vi "FunctionGenerator_Add_Value.vi"(9 "Y Value":dbl, 10 "X Value":dbl, 11 "in FUNCTION_GENERATOR":T1) -> (3 "out FUNCTION_GENERATOR":T1)   [LabVIEW 2019, in "Trajectory_Library.lvlib"]
doc: "Insert new X, Y pair into an existing Function Generator data cluster. If the X values matches an existing X value, the new X and Y values replaces the old values.\n\nInputs:\n - In Function Generator -- Function generator data cluster\n - X -- X value\n - Y -- Y value\n\nOutputs:\n - out Function Generator -- updated data structure"
uses:
  Trajectory_Library.lvlib
  TypeDef/FUNCTION_GENERATOR.ctl
  <vilib>/gmath/NI_Gmath.lvlib
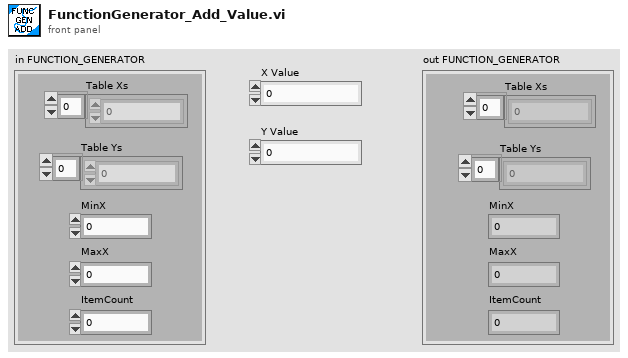
[diagram p1: front panel]
types:
  T1 = typedef "Trajectory_Library.lvlib/FUNCTION_GENERATOR.ctl" = cluster{"Table Xs":dbl[], "Table Ys":dbl[], "MinX":dbl, "MaxX":dbl, "ItemCount":i32}
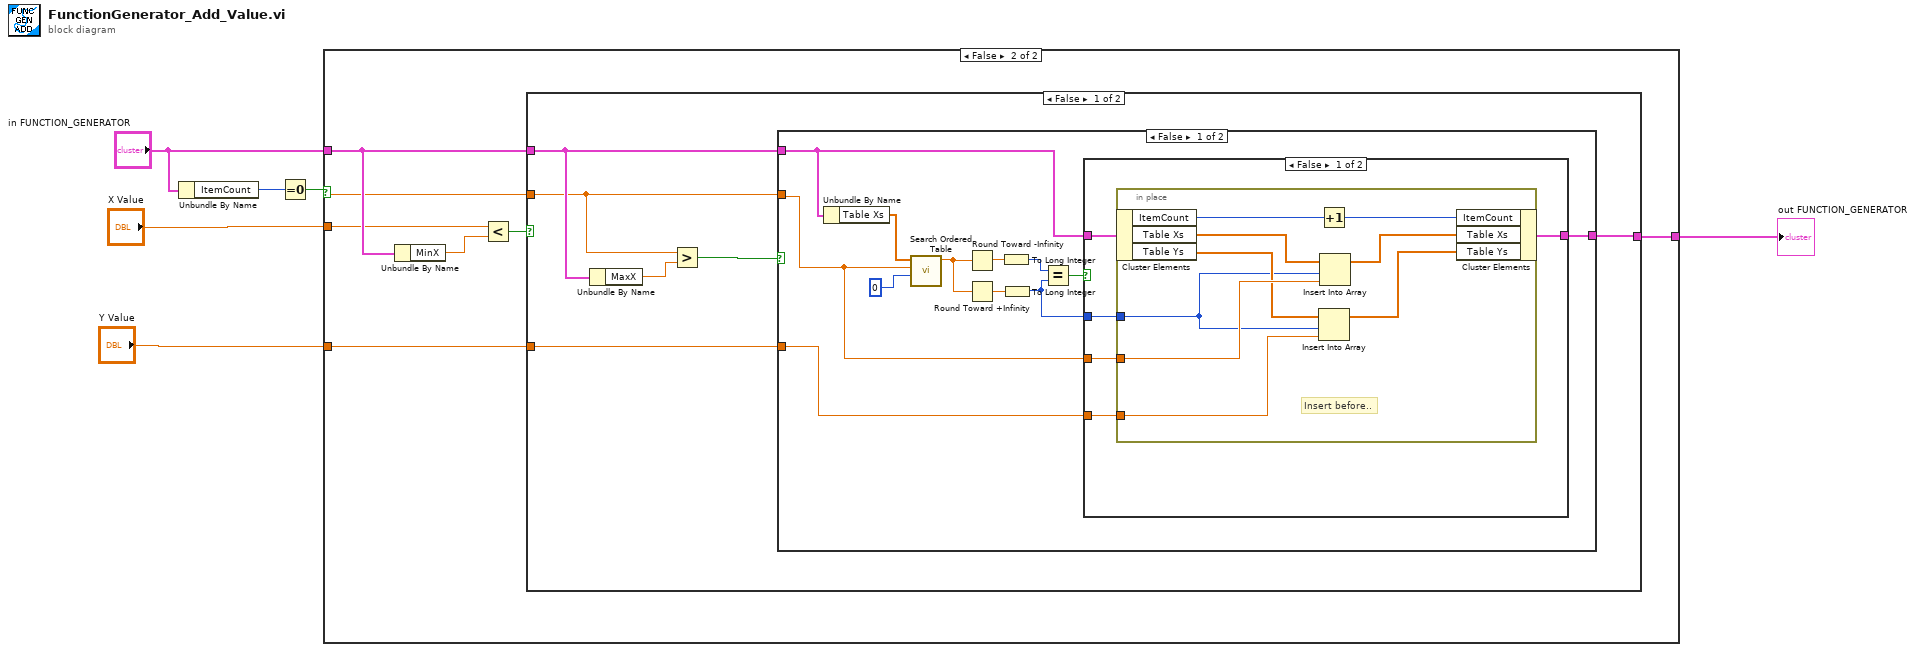
[diagram p0: block diagram]
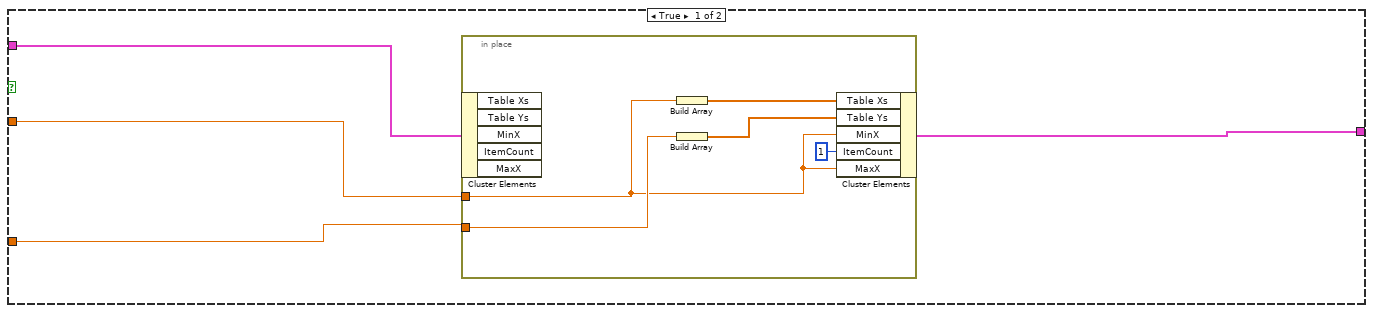
[diagram p2: hidden frame]
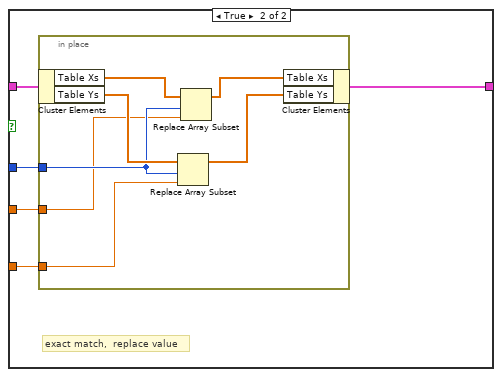
[diagram p3: hidden frame]
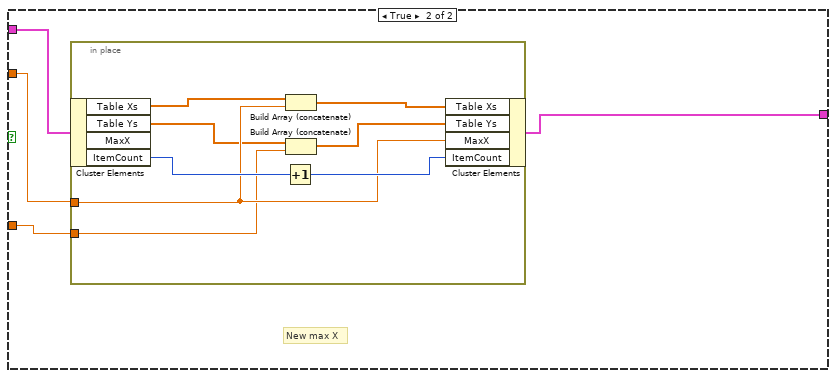
[diagram p4: hidden frame]
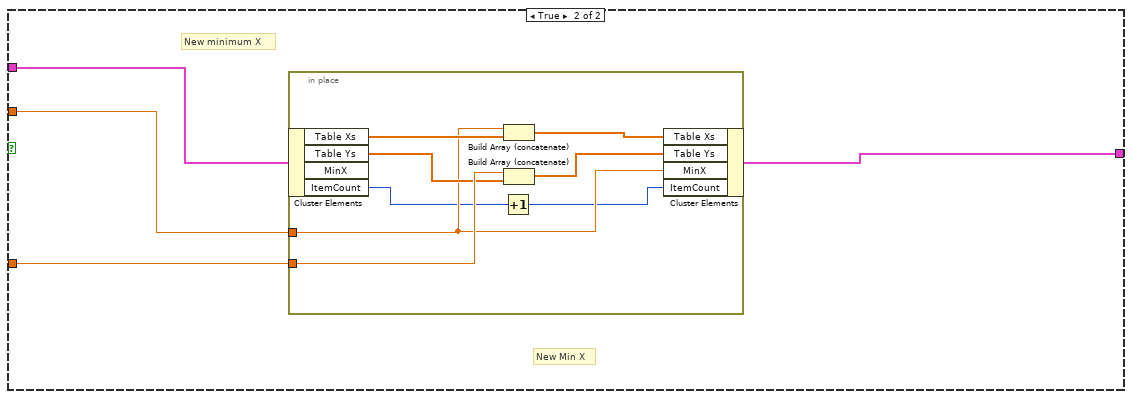
[diagram p5: hidden frame]
diagram:
  n1 = Unbundle By Name("in FUNCTION_GENERATOR") -> ("ItemCount"=w1:i32)
  n2 = Equal To 0?(x=w1) -> (x = 0?=w2:bool)
  n3 = case shown="False" w2 {
    tunnel: "in FUNCTION_GENERATOR" -> [w10 w19]
    tunnel: "X Value" -> [w8 w18]
    tunnel: "Y Value" -> [w7 w17]
    tunnel: [w9 w16] -> w4
    frame True {
      n4 = in-place {
        in-place-border: w8 -> [w12]
        in-place-border: w7 -> [w15]
        n5 = in-place-cluster #1(w10) -> ()  [unwired: 5 out]
        n6 = Build Array(w12) -> (w14:dbl[])
        n7 = Build Array(w15) -> (w13:dbl[])
        n8 = in-place-cluster #1("Table Xs"=w14, "Table Ys"=w13, "MinX"=w12, "ItemCount"=1, "MaxX"=w12) -> (w9:T1)
      }
    }
    frame False {
      n9 = Unbundle By Name(w19) -> ("MinX"=w21:dbl)
      n10 = Less?(x=w18, y=w21) -> (x < y?=w20:bool)
      n11 = case shown="False" w20 {
        tunnel: w19 -> [w26 w81]
        tunnel: w18 -> [w24 w80]
        tunnel: w17 -> [w23 w79]
        tunnel: [w25 w78] -> w16
        frame False {
          n12 = Unbundle By Name(w26) -> ("MaxX"=w27:dbl)
          n13 = Greater?(x=w24, y=w27) -> (0:w22:bool)
          n14 = case shown="False" w22 {
            tunnel: w26 -> [w32 w69]
            tunnel: [w28 w68] -> w25
            tunnel: w24 -> [w30 w67]
            tunnel: w23 -> [w29 w66]
            frame False {
              n15 = Unbundle By Name(w32) -> ("Table Xs"=w38:dbl[])
              n16 = call <vilib>:"Search Ordered Table.vi"("starting index"=0, "x value"=w30, "ordered x array"=w38) -> ("fractional index"=w37:dbl)  [unwired: 8 in]
              n17 = Round Toward -Infinity(1:w37) -> (0:w35:dbl)
              n18 = Round Toward +Infinity(x=w37) -> (ceil(x): smallest int >= x=w36:dbl)
              n19 = To Long Integer(number=w35) -> (32bit integer=w34:i32)
              n20 = To Long Integer(number=w36) -> (32bit integer=w31:i32)
              n21 = Equal?(x=w34, y=w31) -> (x = y?=w33:bool)
              n22 = case shown="False" w33 {
                tunnel: w32 -> [w41 w58]
                tunnel: w31 -> [w44 w57]
                tunnel: w30 -> [w43 w56]
                tunnel: w29 -> [w42 w55]
                tunnel: [w40 w54] -> w28
                frame False {
                  n23 = in-place {
                    in-place-border: w44 -> [w48]
                    in-place-border: w43 -> [w50]
                    in-place-border: w42 -> [w47]
                    # "Insert before.."
                    n24 = in-place-cluster #2(w41) -> ("ItemCount"=w53:i32, "Table Xs"=w51:dbl[], "Table Ys"=w49:dbl[])
                    n25 = Increment(x=w53) -> (x+1=w52:i32)
                    n26 = Insert Into Array(array=w49, index=w48, new element=w47) -> (w45:dbl[])
                    n27 = Insert Into Array(array=w51, index=w48, new element=w50) -> (w46:dbl[])
                    n28 = in-place-cluster #2("ItemCount"=w52, "Table Xs"=w46, "Table Ys"=w45) -> (w40:T1)
                  }
                }
                frame True {
                  # "exact match,  replace value"
                  n29 = in-place {
                    in-place-border: w57 -> [w63]
                    in-place-border: w56 -> [w62]
                    in-place-border: w55 -> [w61]
                    n30 = in-place-cluster #3(w58) -> ("Table Xs"=w65:dbl[], "Table Ys"=w64:dbl[])
                    n31 = Replace Array Subset(array=w64, new element=w61, index=w63) -> (w59:dbl[])
                    n32 = Replace Array Subset(array=w65, new element=w62, index=w63) -> (w60:dbl[])
                    n33 = in-place-cluster #3("Table Xs"=w60, "Table Ys"=w59) -> (w54:T1)
                  }
                }
              }
            }
            frame True {
              # "New max X"
              n34 = in-place {
                in-place-border: w67 -> [w73]
                in-place-border: w66 -> [w70]
                n35 = in-place-cluster #4(w69) -> ("Table Xs"=w72:dbl[], "Table Ys"=w71:dbl[], "ItemCount"=w75:i32)  [unwired: 1 out]
                n36 = Increment(x=w75) -> (x+1=w74:i32)
                n37 = Build Array (concatenate)(w72, w73) -> (w77:dbl[])
                n38 = Build Array (concatenate)(w71, w70) -> (w76:dbl[])
                n39 = in-place-cluster #4("Table Xs"=w77, "Table Ys"=w76, "MaxX"=w73, "ItemCount"=w74) -> (w68:T1)
              }
            }
          }
        }
        frame True {
          # "New Min X"
          # "New minimum X"
          n40 = in-place {
            in-place-border: w80 -> [w84]
            in-place-border: w79 -> [w89]
            n41 = in-place-cluster #5(w81) -> ("Table Xs"=w88:dbl[], "Table Ys"=w85:dbl[], "ItemCount"=w83:i32)  [unwired: 1 out]
            n42 = Increment(x=w83) -> (x+1=w82:i32)
            n43 = Build Array (concatenate)(w84, w88) -> (w87:dbl[])
            n44 = Build Array (concatenate)(w89, w85) -> (w86:dbl[])
            n45 = in-place-cluster #5("Table Xs"=w87, "Table Ys"=w86, "MinX"=w84, "ItemCount"=w82) -> (w78:T1)
          }
        }
      }
    }
  }
  "out FUNCTION_GENERATOR" <- w4
